vi "stop listening.vi"(8 "error in":errorcluster, 11 "connection server in":refnum<class "connection server.lvclass">) -> (0 "error out":errorcluster, 3 "connection server out":refnum<class "connection server.lvclass">)   [LabVIEW 2015, in "connection server.lvclass"]
uses:
  connection server.lvclass
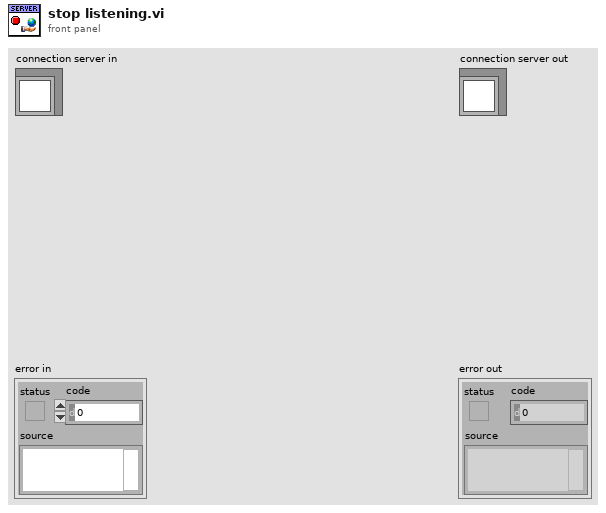
[diagram p1: front panel]
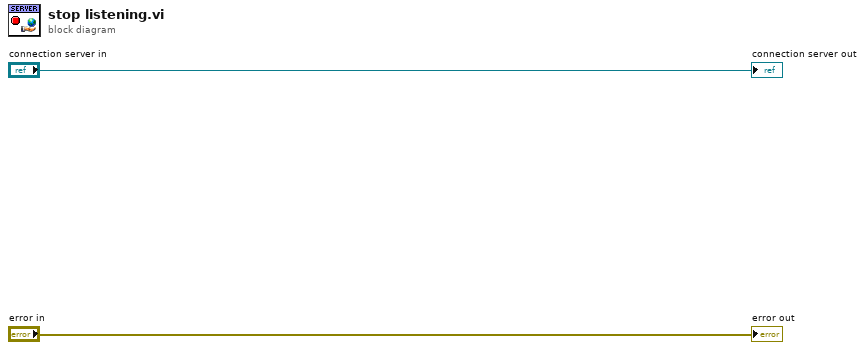
[diagram p0: block diagram]
diagram:
  "error out" <- "error in"
  "connection server out" <- "connection server in"
